vi "4.3.vi"() -> ()   [LabVIEW 2016]
uses:
  <vilib>/measure/NI_MABase.lvlib
panel:
  out "XY图":cluster{"Y":dbl[], "Y":dbl[]}(graph)
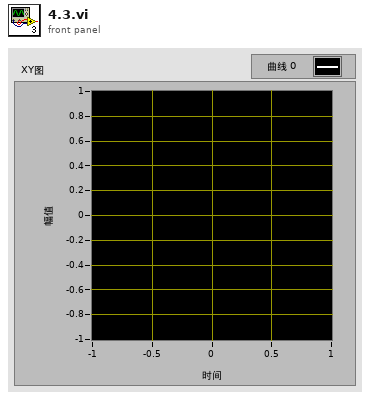
[diagram p1: front panel]
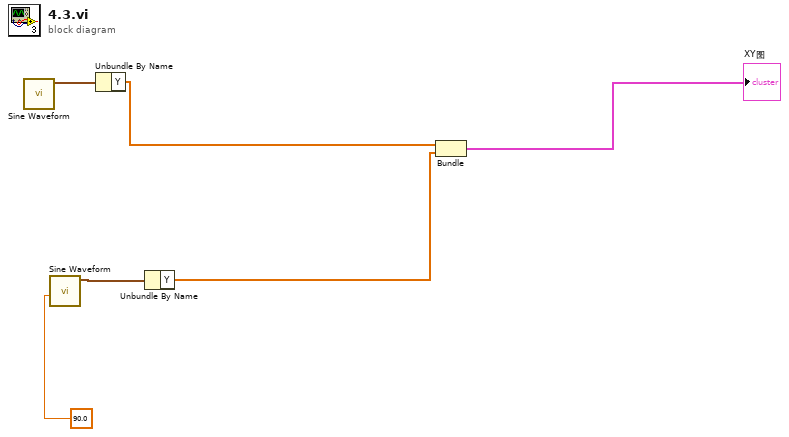
[diagram p0: block diagram]
diagram:
  n1 = call <vilib>:"Sine Waveform.vi"() -> ("signal out"=w6:waveform(dbl))  [unwired: 10 in, 1 out]
  n2 = call <vilib>:"Sine Waveform.vi"("phase"=90.0) -> ("signal out"=w5:waveform(dbl))  [unwired: 9 in, 1 out]
  n3 = Unbundle By Name(w6) -> ("Y"=w3:dbl[])
  n4 = Unbundle By Name(w5) -> ("Y"=w1:dbl[])
  n5 = Bundle("Y"=w3, "Y"=w1) -> (→"XY图":cluster{"Y":dbl[], "Y":dbl[]})  [unwired: 1 in]
